vi "质控关于.vi"(11 "Slave ID":T1) -> ()   [LabVIEW 2016, in "质控单元V1.lvlib"]
panel:
  in  "关闭":bool
  out "固件信息：":string
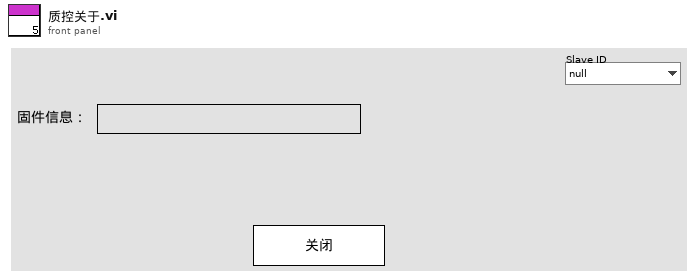
[diagram p1: front panel]
types:
  T1 = typedef "质控单元V1.lvlib/质控slave id.ctl" = enum16{"null", "氨氮", "总磷", "CODMn", "CODCr", "总氮"}
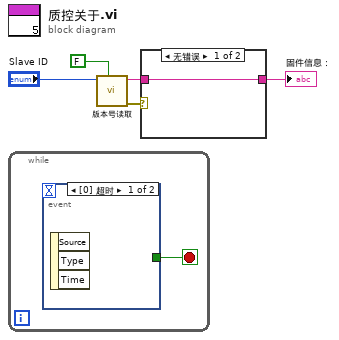
[diagram p0: block diagram]
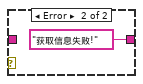
[diagram p2: hidden frame]
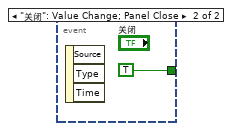
[diagram p3: hidden frame]
diagram:
  n1 = while {
    stop <- w6 stop-if-true
    n2 = event shown="[0] 超时" {
      selector: _ -> [_ _]
      dyn-events: _ -> [_ _]
      timeout: _ -> [_ _]
      tunnel: [_ TRUE] -> w6
      event Timeout {
        n3 = event-data() -> ()  [unwired: 1 in, 3 out]
      }
      event "关闭": Value Change; Panel Close {
        n4 = event-data() -> ()  [unwired: 1 in, 3 out]
      }
    }
  }
  n5 = call "版本号读取.vi"("是否启用通讯通知"=FALSE, "Slave ID"="Slave ID") -> ("error out"=w2:errorcluster, "固件信息"=w3:string)  [unwired: 8 in]
  n6 = case shown="无错误" w2 {
    tunnel: [w8 "获取信息失败!" ("固件信息")] -> w4
    tunnel: w3 -> [w8 _]
    frame No Error {
    }
    frame Error {
    }
  }
  "固件信息：" <- w4
